vi "niRFUtil WFM Apply Phase Offset.vi"(0 "Waveform In":T1 {"y" format="%.2f"; "dx" format="%^.2e"; "x0" format="%^.2e"}, 13 "Offset, degrees":sgl format="%.2f") -> (4 "Waveform Out":T1 {"y" format="%.2f"; "dx" format="%^.2e"; "x0" format="%^.2e"})   [LabVIEW 2015, in "niRFUtil.lvlib"]
doc: "(c) Copyright 2006, National Instruments, Inc. This VI may not be duplicated, sold, or distributed without written consent from National Instruments."
uses:
  niRFUtil.lvlib
  Includes/niRFUtil INC Complex Waveform.ctl
  Includes/niRFUtil INC Complex Array.ctl
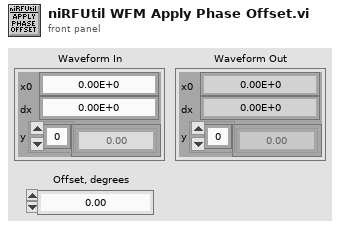
[diagram p1: front panel]
types:
  T1 = typedef "niRFUtil.lvlib/niRFUtil INC Complex Waveform.ctl" = cluster{"x0":dbl, "dx":dbl, "y":T2}
  T2 = typedef "niRFUtil.lvlib/niRFUtil INC Complex Array.ctl" = csg[]
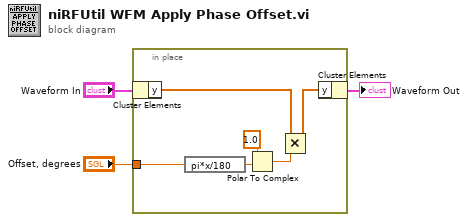
[diagram p0: block diagram]
diagram:
  n1 = in-place {
    in-place-border: "Offset, degrees" -> [w9]
    n2 = in-place-cluster #1("Waveform In") -> ("y"=w5:T2)
    n3 = expression code="pi*x/180"(w9) -> (w8:sgl)
    n4 = Polar To Complex(1:w8, 2:sgl 1.0 ("r")) -> (0:w7:csg)
    n5 = Multiply(x=w5, y=w7) -> (x*y=w4:T2)
    n6 = in-place-cluster #1("y"=w4) -> (→"Waveform Out":T1)
  }
